vi "loadSingleToneData.vi"(8 "error in (no error)":errorcluster, 10 "SingleTone":refnum<class "SingleTone.lvclass">, 11 "SingleToneAction in":refnum<class "SingleToneAction.lvclass">) -> (0 "error out":errorcluster, 2 "SingleTone out":refnum<class "SingleTone.lvclass">, 3 "SingleToneAction out":refnum<class "SingleToneAction.lvclass">)   [LabVIEW 2009, in "Views.lvlib" / "ScriptEditor.lvlib" / "SingleToneAction.lvclass"]
uses:
  SingleToneAction.lvclass
  Tools/Scripting/ScriptingEvent/ScriptEvents/SingleTone/SingleTone.lvclass
  Tools/Scripting/ScriptingEvent/ScriptEvents/SingleToneArray/SingleToneArray.lvclass
  SingleToneAction.lvclass/SingleToneAction.ctl
  Tools/DatabaseHelpers/Database Objects/Channel/Channel.lvclass
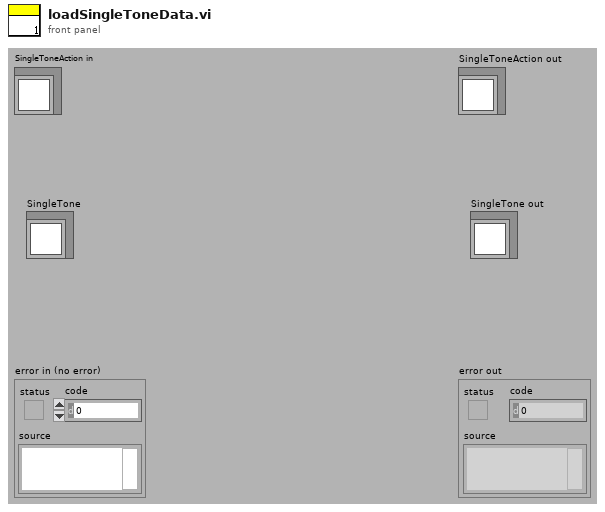
[diagram p1: front panel]
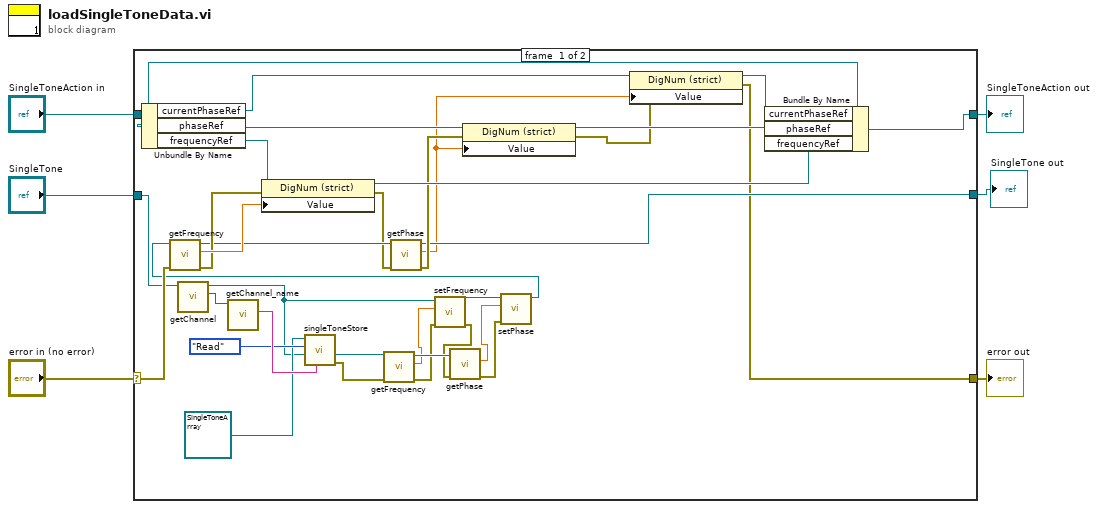
[diagram p0: block diagram]
diagram:
  n1 = case shown="No Error" "error in (no error)" {
    selector: "error in (no error)" -> [w40 w42]
    tunnel: [w21 w42] -> w5
    tunnel: [w38 w41] -> w3
    tunnel: "SingleToneAction in" -> [w39 w41]
    tunnel: "SingleTone" -> [w12 _]
    tunnel: [w30 _] -> w1
    frame #0 {
      n2 = Unbundle By Name(w39) -> ("currentPhaseRef"=w22:refnum<vi>, "phaseRef"=w33:refnum<vi>, "frequencyRef"=w37:refnum<vi>)
      n3 = call-dynamic "getChannel.vi"("ScriptEvent.lvclass in"=w12) -> ("Channel.lvclass"=w28:refnum<class "Channel.lvclass">, "ScriptEvent.lvclass out"=w18:refnum<class "SingleTone.lvclass">)  [unwired: 8 in, 1 out]
      n4 = call "getChannel_name.vi"("Channel.lvclass in"=w28) -> ("channel_name"=w27:string)  [unwired: 8 in, 2 out]
      n5 = call "singleToneStore.vi"("channel_name"=w27, "SingleTone.lvclass"=w18, "action"=enum16{"Write", "Read"}."Read", "SingleToneArray in"=refnum<class "SingleToneArray.lvclass"> refnum) -> ("error out"=w10:errorcluster, "SingleTone.lvclass out"=w17:refnum<class "SingleTone.lvclass">)  [unwired: 4 in, 2 out]
      n6 = call "getFrequency.vi"("error in (no error)"=w10, "SingleTone.lvclass in"=w17) -> ("error out"=w9:errorcluster, "frequency"=w15:dbl, "SingleTone.lvclass out"=w16:refnum<class "SingleTone.lvclass">)  [unwired: 7 in]
      n7 = call "setFrequency.vi"("error in (no error)"=w9, "frequency"=w15, "SingleTone.lvclass in"=w18) -> ("error out"=w8:errorcluster, "SingleTone.lvclass out"=w13:refnum<class "SingleTone.lvclass">)  [unwired: 7 in]
      n8 = call "getPhase.vi"("error in (no error)"=w8, "SingleTone.lvclass in"=w16) -> ("error out"=w7:errorcluster, "phase"=w14:dbl)  [unwired: 7 in, 1 out]
      n9 = call "setPhase.vi"("error in (no error)"=w7, "phase"=w14, "SingleTone.lvclass in"=w13) -> ("SingleTone.lvclass out"=w11:refnum<class "SingleTone.lvclass">)  [unwired: 7 in, 1 out]
      n10 = call "getFrequency.vi"("error in (no error)"=w40, "SingleTone.lvclass in"=w11) -> ("error out"=w35:errorcluster, "frequency"=w36:dbl, "SingleTone.lvclass out"=w29:refnum<class "SingleTone.lvclass">)  [unwired: 7 in]
      n11 = property class="DigNum (strict)"(reference=w37, error in=w35, "Value"=w36) -> (reference out=w34:refnum<vi>, error out=w24:errorcluster)
      n12 = call "getPhase.vi"("error in (no error)"=w24, "SingleTone.lvclass in"=w29) -> ("error out"=w32:errorcluster, "phase"=w19:dbl, "SingleTone.lvclass out"=w30:refnum<class "SingleTone.lvclass">)  [unwired: 7 in]
      n13 = property class="DigNum (strict)"(reference=w33, error in=w32, "Value"=w19) -> (reference out=w31:refnum<vi>, error out=w23:errorcluster)
      n14 = property class="DigNum (strict)"(reference=w22, error in=w23, "Value"=w19) -> (reference out=w20:refnum<vi>, error out=w21:errorcluster)
      n15 = Bundle By Name(cluster=w39, "currentPhaseRef"=w20, "phaseRef"=w31, "frequencyRef"=w34) -> (w38:refnum<class "SingleToneAction.lvclass">)
    }
    frame #1 {
    }
  }
  "error out" <- w5
  "SingleToneAction out" <- w3
  "SingleTone out" <- w1
